vi "Send Command (non-enum).vi"(8 "error in (no error)":errorcluster, 10 "Commands":string[](array[string]), 11 "Gen 2 in":refnum<class "Gen 2.lvclass">) -> (0 "error out":errorcluster, 3 "Gen 2 out":refnum<class "Gen 2.lvclass">)   [LabVIEW 2018, in "Gen 2.lvlib" / "Gen 2.lvclass"]
doc: "This Override can send multiple commands that do not require a response from the targeted device."
uses:
  Gen 2.lvclass
  PPLs/Laser/Parent/Laser.lvlibp/Laser.lvclass
  C:/Projects/LabVIEW/PPLs/Laser/Parent/Laser.lvlibp/Laser.lvclass
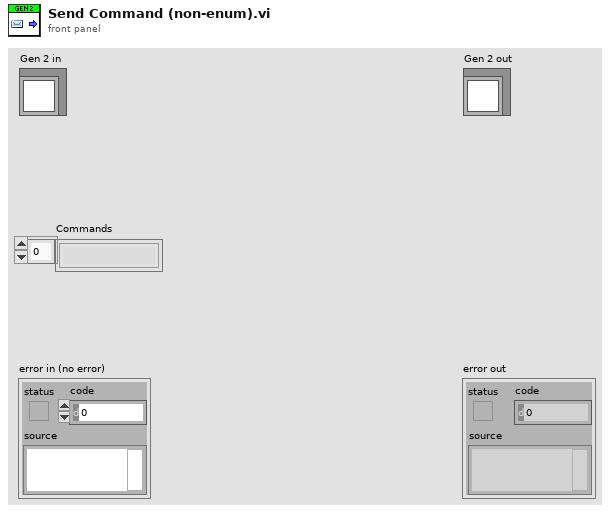
[diagram p1: front panel]
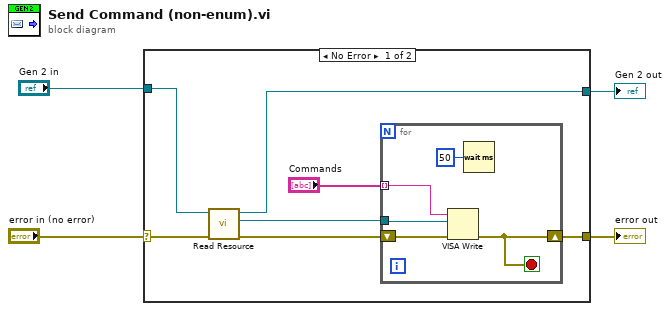
[diagram p0: block diagram]
diagram:
  n1 = case shown="No Error" "error in (no error)" {
    selector: "error in (no error)" -> [w11 w17]
    tunnel: "Gen 2 in" -> [w10 w18]
    tunnel: [w6 w18] -> w2
    tunnel: [w5 w17] -> w1
    frame No Error {
      n2 = call "Read Resource.vi"("error in (no error)"=w11, "Laser in"=w10) -> ("error out"=w9:errorcluster, "Resource"=w8:refnum<visa-resource-name>, "Laser out"=w6:refnum<class "Gen 2.lvclass">)  [unwired: 7 in]
      n3 = for {
        shift-right: [w12] -> w5
        shift-left: w9 -> [w14]
        tunnel: w8 -> [w16]
        tunnel: "Commands" -> [w15] mode=indexing
        stop <- w12 stop-if-true
        n4 = VISA Write(VISA resource name=w16, write buffer=w15, error in (no error)=w14) -> (error out=w12:errorcluster)  [unwired: 2 out]
        n5 = Wait (ms)(milliseconds to wait=u32 50) -> ()  [unwired: 1 out]
      }
    }
    frame Error {
    }
  }
  "error out" <- w1
  "Gen 2 out" <- w2
